vi "FPGA_SinglePointSuspension.vi"() -> ()   [LabVIEW 2024]
uses:
  <vilib>/rvi/FXPMathLib/FxpDiv/subVIs/nifxpmath_Div_SimConfig.ctl
  <vilib>/rvi/Emulation/niFpgaGetClockAttributes.vi
  <vilib>/rvi/Emulation/niFpgaSctlEmulationGetInTimedLoop.vi
  <vilib>/rvi/Emulation/niFpgaEmulationReportErrorSimple.vi
  <vilib>/rvi/Emulation/niFpgaEmulationIsFPGAContextNoSignature.vi
  <vilib>/rvi/DataTransferAndStorage/Container/Common/niFpgaContainerGetUniqueNameForEmu.vi
  <vilib>/rvi/Memory/Memory_Emulation/niFpgaMemoryEmulationCacheClearOnFirstRun.vi
  <vilib>/rvi/Memory/Memory_Emulation/nirvimemoryEmulationManagerCache_MakeExclusive.vi
  <vilib>/rvi/Memory/Memory_Emulation/niFpgaMemoryEmulationValidateCache.vi
  <vilib>/rvi/Memory/Memory_Emulation/nirvimemoryEmulationManagerCache_InsertValue.vi
  <vilib>/Utility/error.llb/Clear Errors.vi
  <vilib>/rvi/Memory/Memory_Emulation/nirvimemoryEmulationManagerCache_ReleaseExclusive.vi
  <vilib>/rvi/Memory/Memory_Emulation/nirvimemoryEmulationManagerCache_GetValue.vi
  <vilib>/rvi/Memory/Memory_Emulation/nirvimemoryEmulationManagerCache_SetValue.vi
  <vilib>/rvi/Emulation/niFpgaProcessEmulError.vi
  <vilib>/rvi/Emulation/niFpgaCriticalErrorInLSC.vi
  <vilib>/rvi/eio/common/nirviEmuTemplateMethod_errors.vi
  <vilib>/rvi/FXPMathLib/FxpDiv/simVIs/DllFxpDivTemp_sub.vi
  <vilib>/rvi/DataTransferAndStorage/Container/XNode/niFpgaContainer.xnode
  <vilib>/rvi/DataTransferAndStorage/Register/Emulation/niFpgaRegisterEmulation.vi
  <vilib>/eio/EIONode/EIONode.xnode
  <vilib>/rvi/FXPMathLib/FxpAdd/XNode/nifxpmath_Add.xnode
  <vilib>/rvi/FXPMathLib/FxpDiv/XNode/nifxpmath_Div.xnode
  <vilib>/rvi/FXPMathLib/FxpMul/XNode/nifxpmath_Multiplier.xnode
  <vilib>/rvi/FXPMathLib/FxpSub/XNode/nifxpmath_Sub.xnode
  <vilib>/rvi/FXPMathLib/sim/FxpSim.dll
panel:
  in  "stop":bool
  in  "RetRate us":i32
  in  "AppRate us":i32
  in  "Retract":fxp<+/-,48,16>
  in  "Y":fxp<+/-,48,16>
  in  "X":fxp<+/-,48,16>
  in  "Threshold":fxp<+/-,48,16>
  out "TargetDone?":bool
  out "ScanFinished?":bool
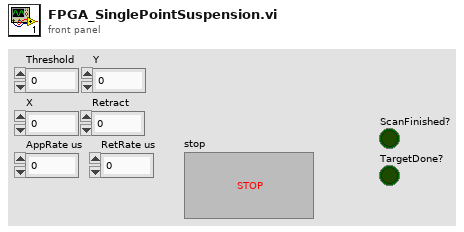
[diagram p1: front panel]
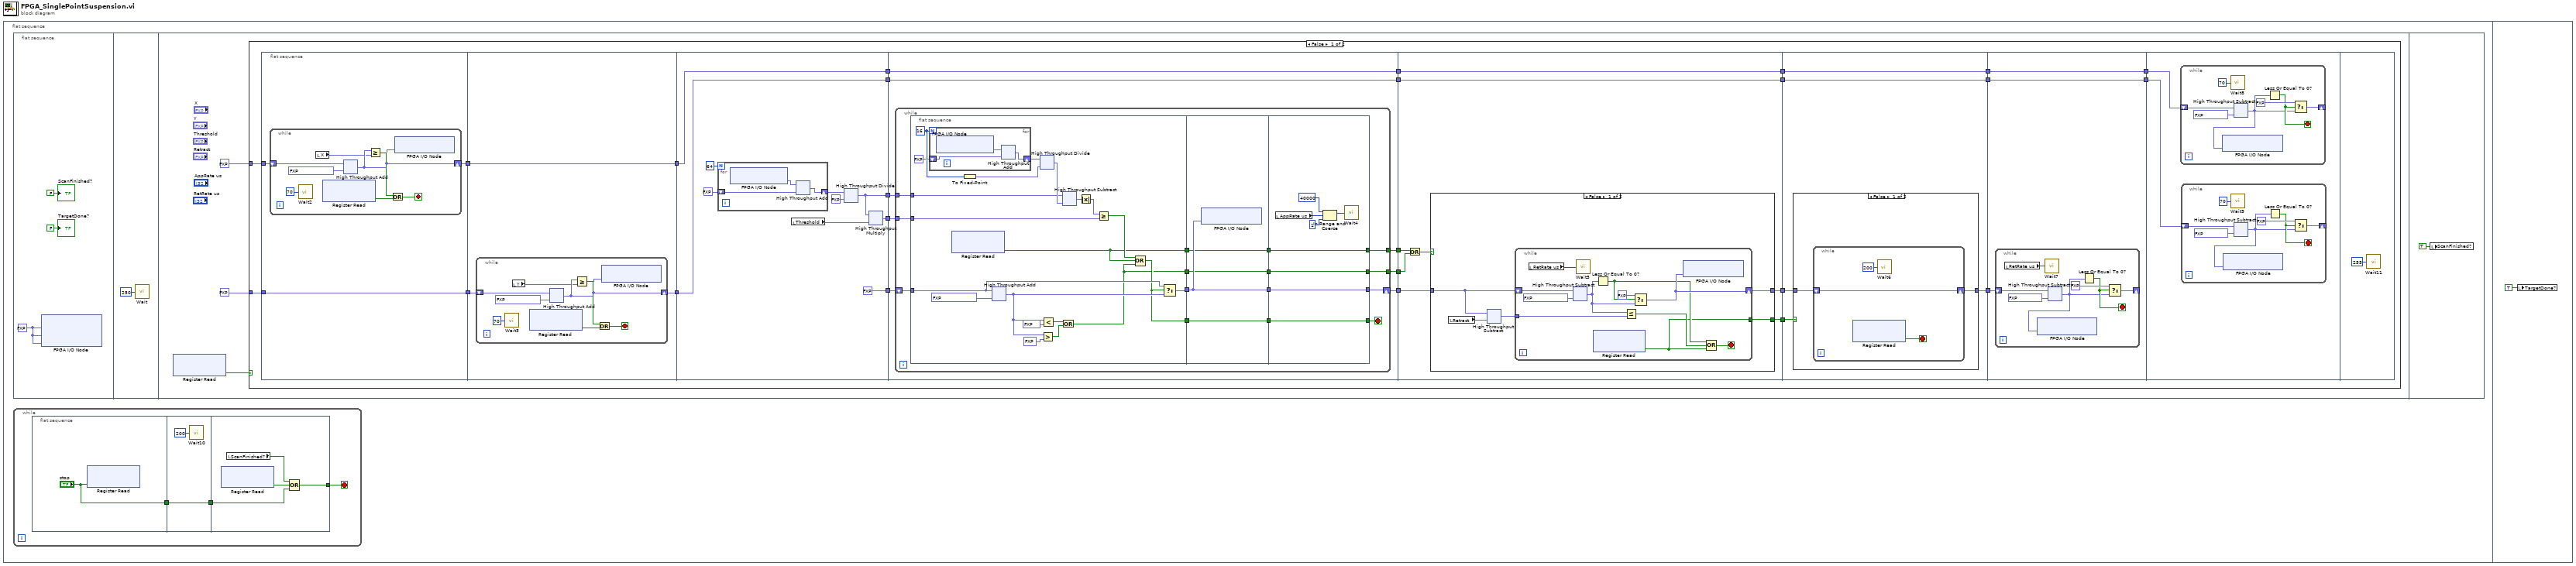
[diagram p0: block diagram]
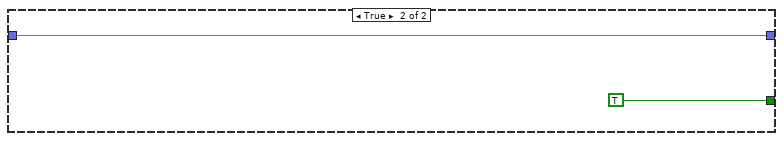
[diagram p2: hidden frame]
diagram:
  n1 = flat-sequence {
    frame #0 {
      n2 = flat-sequence {
        frame #0 {
          w13 = fxp<+/-,20,5> 0.0 ("Connector0/AO0")
          n3 = xnode "FPGA I/O Node"("Connector0/AO0"=w13, "Connector0/AO1"=w13, "Connector0/AO2"=w13) -> ()  [unwired: 3 in, 3 out]
          "ScanFinished?" <- FALSE
          "TargetDone?" <- FALSE
        }
        frame #1 {
          n4 = call "Wait"("Count(mSec)"=u8 250) -> ()  [unwired: 1 out]
        }
        frame #2 {
          n5 = xnode ("Register Read")() -> ("Data"=w17:bool)  [unwired: 1 in, 1 out]
          n6 = case shown="False" w17 {
            tunnel: fxp<+/-,48,16> 0.0 ("Y") -> [w42 _]
            tunnel: fxp<+/-,48,16> 0.0 ("Y") -> [w40 _]
            frame False {
              n7 = flat-sequence {
                tunnel: w42 -> [w45]
                tunnel: [w44] -> w41
                tunnel: w40 -> [w43]
                tunnel: [w43] -> w39
                tunnel: w41 -> [w54]
                tunnel: w39 -> [w56]
                tunnel: [w55] -> w29
                tunnel: [w54] -> w28
                tunnel: [w69] -> w38
                tunnel: [w68] -> w37
                tunnel: [fxp<+/-,48,16> 0.0] -> w36
                tunnel: w29 -> [w65]
                tunnel: w28 -> [w66]
                tunnel: [w66] -> w27
                tunnel: [w65] -> w26
                tunnel: w38 -> [w112]
                tunnel: w37 -> [w111]
                tunnel: w36 -> [w110]
                tunnel: [w109] -> w35
                tunnel: [w108] -> w34
                tunnel: [w107] -> w33
                tunnel: w27 -> [w106]
                tunnel: w26 -> [w105]
                tunnel: [w106] -> w25
                tunnel: [w105] -> w24
                tunnel: w35 -> [w198]
                tunnel: w34 -> [w197]
                tunnel: w33 -> [w195]
                tunnel: [w194] -> w32
                tunnel: [w193] -> w31
                tunnel: w25 -> [w192]
                tunnel: w24 -> [w191]
                tunnel: [w192] -> w23
                tunnel: [w191] -> w22
                tunnel: w32 -> [w221]
                tunnel: w31 -> [w220]
                tunnel: [w219] -> w30
                tunnel: w23 -> [w218]
                tunnel: w22 -> [w217]
                tunnel: [w218] -> w20
                tunnel: [w217] -> w19
                tunnel: w30 -> [w230]
                tunnel: [w229] -> w21
                tunnel: w20 -> [w229]
                tunnel: w19 -> [w228]
                tunnel: [w228] -> w18
                tunnel: w21 -> [w239]
                tunnel: w18 -> [w238]
                frame #0 {
                  n8 = while {
                    shift-right: [w48] -> w44
                    shift-left: w45 -> [w50]
                    stop <- w51 stop-if-true
                    n9 = call "Wait2"("Count(uSec)"=u32 70) -> ()  [unwired: 1 out]
                    n10 = local read "X"() -> (w46:fxp<+/-,48,16>)
                    n11 = xnode ("Register Read")() -> ("Data"=w52:bool)  [unwired: 1 in, 1 out]
                    n12 = xnode ("High Throughput Add")("x"=w50, "y"=fxp<+/-,48,16> 0.00030517578125) -> ("x+y"=w48:fxp<+/-,48,16>)
                    n13 = Greater Or Equal?(x=w48, y=w46) -> (x >= y?=w49:bool)
                    n14 = Or(x=w49, y=w52) -> (x .or. y?=w51:bool)
                    n15 = xnode "FPGA I/O Node"("Connector0/AO0"=w48) -> ()  [unwired: 1 in, 1 out]
                  }
                }
                frame #1 {
                  n16 = while {
                    shift-right: [w59] -> w55
                    shift-left: w56 -> [w61]
                    stop <- w62 stop-if-true
                    n17 = call "Wait3"("Count(uSec)"=u32 70) -> ()  [unwired: 1 out]
                    n18 = local read "Y"() -> (w57:fxp<+/-,48,16>)
                    n19 = xnode ("Register Read")() -> ("Data"=w63:bool)  [unwired: 1 in, 1 out]
                    n20 = xnode ("High Throughput Add")("x"=w61, "y"=fxp<+/-,48,16> 0.00030517578125) -> ("x+y"=w59:fxp<+/-,48,16>)
                    n21 = Greater Or Equal?(x=w59, y=w57) -> (x >= y?=w60:bool)
                    n22 = Or(x=w60, y=w63) -> (x .or. y?=w62:bool)
                    n23 = xnode "FPGA I/O Node"("Connector0/AO1"=w59) -> ()  [unwired: 1 in, 1 out]
                  }
                }
                frame #2 {
                  n24 = for {
                    N: 64 -> [_]
                    shift-right: [w102] -> w71
                    shift-left: fxp<+/-,48,16> 0.0 -> [w103]
                    n25 = xnode "FPGA I/O Node"() -> ("Connector0/AI3"=w104:fxp<+/-,27,5>)  [unwired: 1 in, 1 out]
                    n26 = xnode ("High Throughput Add")("x"=w104, "y"=w103) -> ("x+y"=w102:fxp<+/-,48,16>)
                  }
                  n27 = local read "Threshold"() -> (w70:fxp<+/-,48,16>)
                  n28 = xnode "High Throughput Divide"("x"=w71, "y"=fxp<+/-,48,16> 64.0) -> ("x/y"=w69:fxp<+/-,48,16>)
                  n29 = xnode ("High Throughput Multiply")("x"=w69, "y"=w70) -> ("x*y"=w68:fxp<+/-,48,16>)
                }
                frame #3 {
                  n30 = while {
                    tunnel: w112 -> [w127]
                    tunnel: w111 -> [w126]
                    shift-right: [w122] -> w107
                    shift-left: w110 -> [w125]
                    tunnel: [w114] -> w109
                    tunnel: [w113] -> w108
                    stop <- w119 stop-if-true
                    n31 = flat-sequence {
                      tunnel: w127 -> [w143]
                      tunnel: w126 -> [w140]
                      tunnel: w125 -> [w133]
                      tunnel: [w131] -> w124
                      tunnel: [w130] -> w121
                      tunnel: [w129] -> w118
                      tunnel: [w128] -> w116
                      tunnel: w124 -> [w182]
                      tunnel: [w182] -> w123
                      tunnel: w121 -> [w181]
                      tunnel: [w181] -> w120
                      tunnel: w118 -> [w180]
                      tunnel: [w180] -> w117
                      tunnel: w116 -> [w179]
                      tunnel: [w179] -> w115
                      tunnel: w123 -> [w186]
                      tunnel: [w186] -> w122
                      tunnel: w120 -> [w185]
                      tunnel: [w185] -> w119
                      tunnel: w117 -> [w184]
                      tunnel: w115 -> [w183]
                      tunnel: [w184] -> w114
                      tunnel: [w183] -> w113
                      frame #0 {
                        w146 = 16
                        n32 = for {
                          N: w146 -> [_]
                          shift-right: [w176] -> w147
                          shift-left: fxp<+/-,48,16> 0.0 -> [w177]
                          n33 = xnode "FPGA I/O Node"() -> ("Connector0/AI3"=w178:fxp<+/-,27,5>)  [unwired: 1 in, 1 out]
                          n34 = xnode ("High Throughput Add")("x"=w178, "y"=w177) -> ("x+y"=w176:fxp<+/-,48,16>)
                        }
                        n35 = xnode ("Register Read")() -> ("Data"=w129:bool)  [unwired: 1 in, 1 out]
                        n36 = To Fixed-Point(number=w146) -> (fixed-point=w145:fxp<+/-,48,16>)  [unwired: 1 in]
                        n37 = xnode ("High Throughput Add")("x"=w133, "y"=fxp<+/-,48,16> 0.00030517578125) -> ("x+y"=w132:fxp<+/-,48,16>)
                        n38 = xnode "High Throughput Divide"("x"=w147, "y"=w145) -> ("x/y"=w144:fxp<+/-,48,16>)
                        n39 = Greater?(x=w132, y=fxp<+/-,48,16> 9.75) -> (0:w136:bool)
                        n40 = Less?(x=w132, y=fxp<+/-,48,16> -0.125) -> (x < y?=w137:bool)
                        n41 = Or(x=w137, y=w136) -> (x .or. y?=w128:bool)
                        n42 = xnode "High Throughput Subtract"("x"=w143, "y"=w144) -> ("x-y"=w142:fxp<+/-,48,16>)
                        n43 = Absolute Value(x=w142) -> (abs(x)=w141:fxp<+,48,16>)
                        n44 = Greater Or Equal?(x=w141, y=w140) -> (x >= y?=w134:bool)
                        n45 = Compound Arithmetic op=OR(w134, w129, w128) -> (w130:bool)
                        n46 = Select(t=w133, s=w130, f=w132) -> (s? t:f=w131:fxp<+/-,48,16>)
                      }
                      frame #1 {
                        n47 = xnode "FPGA I/O Node"("Connector0/AO2"=w182) -> ()  [unwired: 1 in, 1 out]
                      }
                      frame #2 {
                        n48 = local read "AppRate us"() -> (w187:i32)
                        n49 = In Range and Coerce(upper limit=40000, x=w187, lower limit=1) -> (coerced(x)=w190:i32)  [unwired: 1 out]
                        n50 = call "Wait4"("Count(uSec)"=w190) -> ()  [unwired: 1 out]
                      }
                    }
                  }
                }
                frame #4 {
                  n51 = Or(x=w198, y=w197) -> (x .or. y?=w196:bool)
                  n52 = case shown="False" w196 {
                    tunnel: w195 -> [w202 w215]
                    tunnel: [w200 TRUE ("Data")] -> w194
                    tunnel: [w199 w215] -> w193
                    frame False {
                      n53 = local read "Retract"() -> (w203:fxp<+/-,48,16>)
                      n54 = xnode "High Throughput Subtract"("x"=w202, "y"=w203) -> ("x-y"=w201:fxp<+/-,48,16>)
                      n55 = while {
                        tunnel: w201 -> [w212]
                        shift-right: [w209] -> w199
                        shift-left: w202 -> [w214]
                        tunnel: [w205] -> w200
                        stop <- w206 stop-if-true
                        n56 = local read "RetRate us"() -> (w204:i32)
                        n57 = xnode "High Throughput Subtract"("x"=w214, "y"=fxp<+/-,48,16> 0.00030517578125) -> ("x-y"=w211:fxp<+/-,48,16>)
                        n58 = call "Wait5"("Count(uSec)"=w204) -> ()  [unwired: 1 out]
                        n59 = xnode ("Register Read")() -> ("Data"=w205:bool)  [unwired: 1 in, 1 out]
                        n60 = Less Or Equal To 0?(x=w211) -> (x <= 0?=w208:bool)
                        n61 = Less Or Equal?(x=w211, y=w212) -> (x <= y?=w207:bool)
                        n62 = Select(t=fxp<+/-,48,16> 0.0, s=w208, f=w211) -> (s? t:f=w209:fxp<+/-,48,16>)
                        n63 = xnode "FPGA I/O Node"("Connector0/AO2"=w209) -> ()  [unwired: 1 in, 1 out]
                        n64 = Compound Arithmetic op=OR(w208, w207, w205) -> (w206:bool)
                      }
                    }
                    frame True {
                    }
                  }
                }
                frame #5 {
                  n65 = case shown="False" w221 {
                    tunnel: w220 -> [w223 w227]
                    tunnel: [w222 w227] -> w219
                    frame False {
                      n66 = while {
                        shift-right: [w226] -> w222
                        shift-left: w223 -> [w226]
                        stop <- w224 stop-if-true
                        n67 = xnode ("Register Read")() -> ("Data"=w224:bool)  [unwired: 1 in, 1 out]
                        n68 = call "Wait6"("Count(uSec)"=u8 200) -> ()  [unwired: 1 out]
                      }
                    }
                    frame True {
                    }
                  }
                }
                frame #6 {
                  n69 = while {
                    shift-right: [w234] -> _
                    shift-left: w230 -> [w237]
                    stop <- w233 stop-if-true
                    n70 = local read "RetRate us"() -> (w232:i32)
                    n71 = call "Wait7"("Count(uSec)"=w232) -> ()  [unwired: 1 out]
                    n72 = xnode "High Throughput Subtract"("x"=w237, "y"=fxp<+/-,48,16> 0.0048828125) -> ("x-y"=w231:fxp<+/-,48,16>)
                    n73 = xnode "FPGA I/O Node"("Connector0/AO2"=w231) -> ()  [unwired: 1 in, 1 out]
                    n74 = Less Or Equal To 0?(x=w231) -> (x <= 0?=w233:bool)
                    n75 = Select(t=fxp<+/-,48,16> 0.0, s=w233, f=w231) -> (s? t:f=w234:fxp<+/-,48,16>)
                  }
                }
                frame #7 {
                  n76 = while {
                    shift-right: [w250] -> _
                    shift-left: w239 -> [w253]
                    stop <- w249 stop-if-true
                    n77 = call "Wait8"("Count(uSec)"=u32 70) -> ()  [unwired: 1 out]
                    n78 = xnode "High Throughput Subtract"("x"=w253, "y"=fxp<+/-,48,16> 0.0048828125) -> ("x-y"=w248:fxp<+/-,48,16>)
                    n79 = xnode "FPGA I/O Node"("Connector0/AO0"=w248) -> ()  [unwired: 1 in, 1 out]
                    n80 = Less Or Equal To 0?(x=w248) -> (x <= 0?=w249:bool)
                    n81 = Select(t=fxp<+/-,48,16> 0.0, s=w249, f=w248) -> (s? t:f=w250:fxp<+/-,48,16>)
                  }
                  n82 = while {
                    shift-right: [w243] -> _
                    shift-left: w238 -> [w246]
                    stop <- w242 stop-if-true
                    n83 = call "Wait9"("Count(uSec)"=u32 70) -> ()  [unwired: 1 out]
                    n84 = xnode "High Throughput Subtract"("x"=w246, "y"=fxp<+/-,48,16> 0.0048828125) -> ("x-y"=w241:fxp<+/-,48,16>)
                    n85 = xnode "FPGA I/O Node"("Connector0/AO1"=w241) -> ()  [unwired: 1 in, 1 out]
                    n86 = Less Or Equal To 0?(x=w241) -> (x <= 0?=w242:bool)
                    n87 = Select(t=fxp<+/-,48,16> 0.0, s=w242, f=w241) -> (s? t:f=w243:fxp<+/-,48,16>)
                  }
                }
                frame #8 {
                  n88 = call "Wait11"("Count(uSec)"=u8 255) -> ()  [unwired: 1 out]
                }
              }
            }
            frame True {
            }
          }
        }
        frame #3 {
          n89 = local write "ScanFinished?"(TRUE ("ScanFinished?")) -> ()
        }
      }
      n90 = while {
        stop <- w1 stop-if-true
        n91 = flat-sequence {
          tunnel: ["stop"] -> w2
          tunnel: [w5] -> w3
          tunnel: w2 -> [w5]
          tunnel: w3 -> [w8]
          tunnel: [w7] -> w1
          frame #0 {
            n92 = xnode ("Register Read")("Data"="stop") -> ()  [unwired: 1 in, 1 out]
          }
          frame #1 {
            n93 = call "Wait10"("Count(uSec)"=u8 200) -> ()  [unwired: 1 out]
          }
          frame #2 {
            n94 = xnode ("Register Read")() -> ("Data"=w10:bool)  [unwired: 1 in, 1 out]
            n95 = local read "ScanFinished?"() -> (w9:bool)
            n96 = Compound Arithmetic op=OR(w9, w10, w8) -> (w7:bool)
          }
        }
      }
    }
    frame #1 {
      n97 = local write "TargetDone?"(TRUE ("ScanFinished?")) -> ()
    }
  }
